vi "Files_Unable_to_Update.vi"(1 "error in (no error)":errorcluster, 2 "Target Path":path, 3 "Source Path":path) -> ()   [LabVIEW 2018]
uses:
  Globals/Constants_global.vi
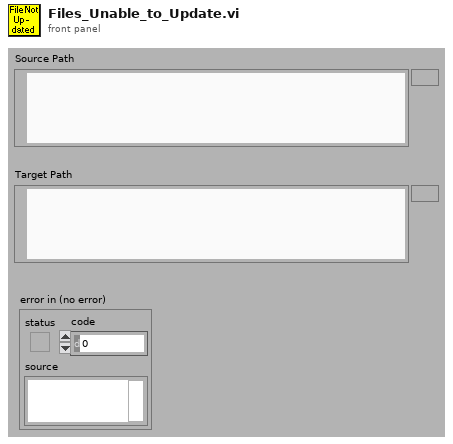
[diagram p1: front panel]
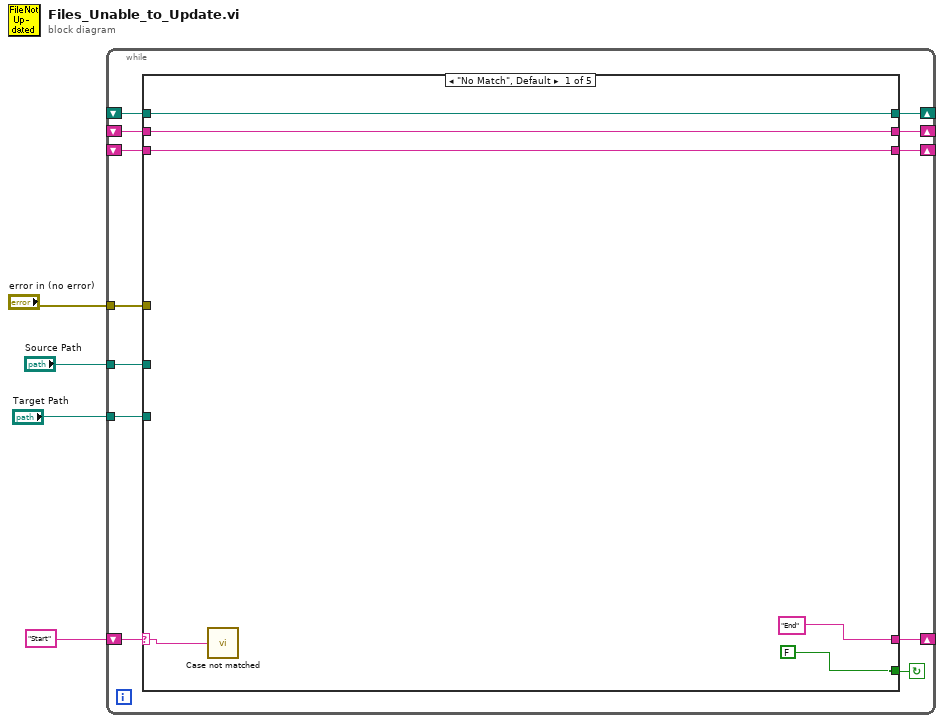
[diagram p0: block diagram]
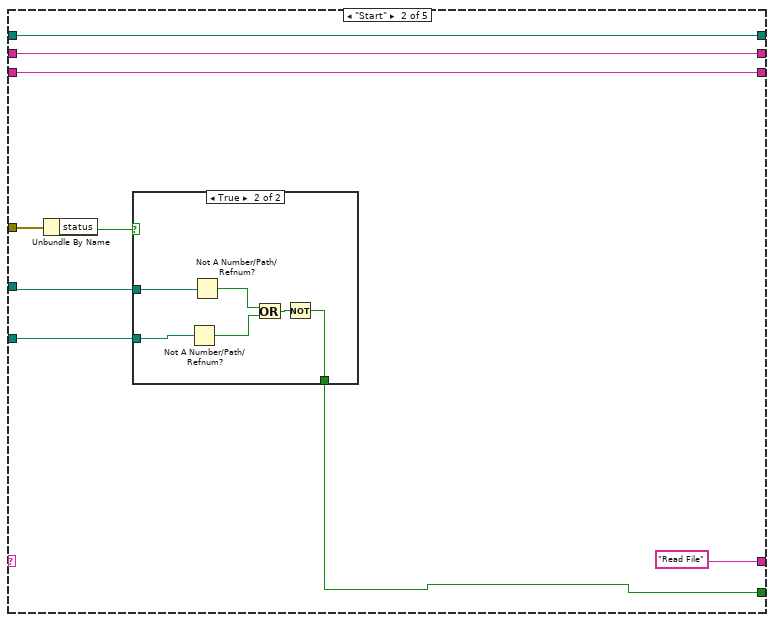
[diagram p2: hidden frame]
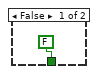
[diagram p3: hidden frame]
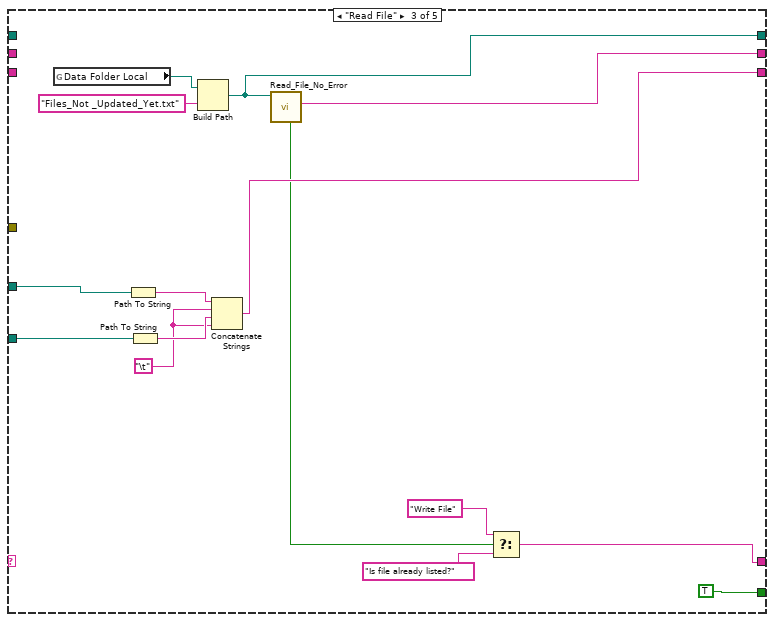
[diagram p4: hidden frame]
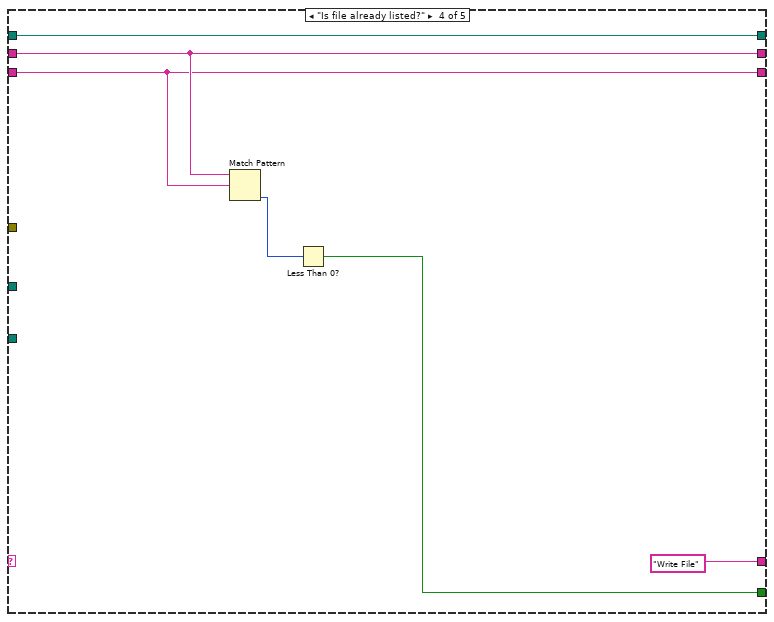
[diagram p5: hidden frame]
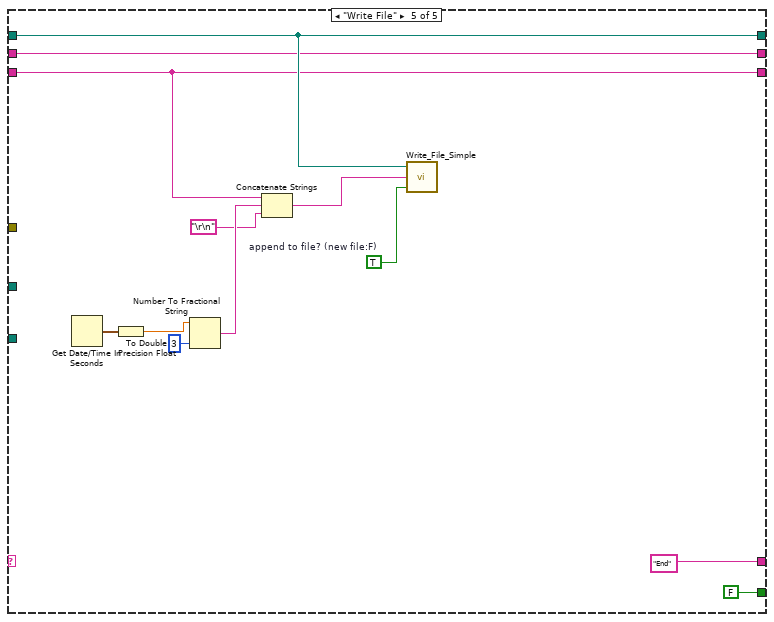
[diagram p6: hidden frame]
diagram:
  n1 = while {
    shift-left: "Start" -> [w14]
    shift-right: [w15] -> _
    tunnel: "error in (no error)" -> [w13]
    shift-right: [w12] -> _
    shift-left: _ -> [w10]
    shift-right: [w11] -> _
    shift-left: _ -> [w9]
    shift-right: [w8] -> _
    shift-left: _ -> [w7]
    tunnel: "Source Path" -> [w6]
    tunnel: "Target Path" -> [w5]
    stop <- w16 continue-if-true
    n2 = case shown="\"No Match\", Default" w14 {
      selector: w14 -> [w17 _ _ _ _]
      tunnel: [FALSE w23 TRUE w57 FALSE ("status")] -> w16
      tunnel: ["End" "Read File" w41 "Write File" "End"] -> w15
      tunnel: w13 -> [_ w30 _ _ _]
      tunnel: [w20 w29 w50 w54 w70] -> w12
      tunnel: [w19 w28 w46 w56 w69] -> w11
      tunnel: w10 -> [w20 w29 _ w54 w70]
      tunnel: w9 -> [w19 w28 _ w56 w69]
      tunnel: [w18 w27 w45 w55 w65] -> w8
      tunnel: w7 -> [w18 w27 _ w55 w65]
      tunnel: w6 -> [_ w25 w40 _ _]
      tunnel: w5 -> [_ w26 w39 _ _]
      frame "No Match", Default {
        n3 = call "Case not matched.vi"("Case Name not Matched"=w17) -> ()
      }
      frame "Start" {
        n4 = Unbundle By Name(w30) -> ("status"=w24:bool)
        n5 = case shown="True" w24 {
          tunnel: w26 -> [_ w38]
          tunnel: w25 -> [_ w37]
          tunnel: [FALSE w33] -> w23
          frame False {
          }
          frame True {
            n6 = Not A Number/Path/Refnum?(number/path/refnum=w38) -> (NaN/Path/Refnum?=w36:bool)
            n7 = Not A Number/Path/Refnum?(number/path/refnum=w37) -> (NaN/Path/Refnum?=w35:bool)
            n8 = Or(x=w35, y=w36) -> (x .or. y?=w34:bool)
            n9 = Not(x=w34) -> (.not. x?=w33:bool)
          }
        }
      }
      frame "Read File" {
        w47 = "\t"
        n10 = global read "Constants_global.vi" "Data Folder Local"() -> (w52:path)
        n11 = Path To String(path=w40) -> (string=w49:string)
        n12 = Path To String(path=w39) -> (string=w48:string)
        n13 = Build Path(base path=w52, name or relative path="Files_Not _Updated_Yet.txt") -> (appended path=w50:path)
        n14 = Concatenate Strings(w49, w47, w48, w47) -> (w45:string)
        n15 = call "Read_File_No_Error.vi"("Filename"=w50) -> ("Error?"=w44:bool, "string"=w46:string)  [unwired: 2 in, 6 out]
        n16 = Select(t="Write File", s=w44, f="Is file already listed?") -> (s? t:f=w41:string)
      }
      frame "Is file already listed?" {
        n17 = Match Pattern(string=w56, regular expression=w55) -> (offset past match=w58:i32)  [unwired: 4 out]
        n18 = Less Than 0?(x=w58) -> (x < 0?=w57:bool)
      }
      frame "Write File" {
        w61 = TRUE  # append to file? (new file:F)
        n19 = Get Date/Time In Seconds() -> (seconds since 1Jan1904=w68:timestamp)
        n20 = To Double Precision Float(number=w68) -> (double precision float=w67:dbl)
        n21 = Number To Fractional String(number=w67, precision (6)=i16 3) -> (F-format string=w64:string)  [unwired: 2 out]
        n22 = Concatenate Strings(w65, w64, "\r\n") -> (w62:string)
        n23 = call "Write_File_Simple.vi"("append to file? (new file:F)"=w61, "character string"=w62, "file path"=w70) -> ()  [unwired: 2 out]
      }
    }
  }
